vi "TestValid.vi"() -> ()   [LabVIEW 2023, in "HAF.lvlib"]
uses:
  HAF.lvlib
  DriverSetting/DriverSetting.lvclass
panel:
  out "error out":errorcluster
  out "Valid":bool
  out "DriverSetting Out":refnum<class "DriverSetting.lvclass">
  in  "error in (no error) 2":errorcluster
  in  "Type":string
  in  "DriverSetting In":refnum<class "DriverSetting.lvclass">
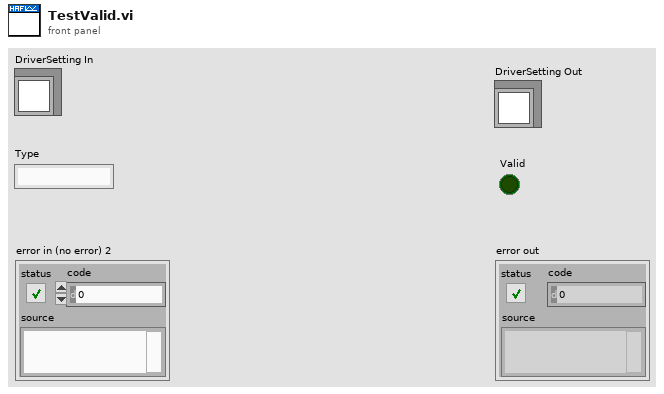
[diagram p1: front panel]
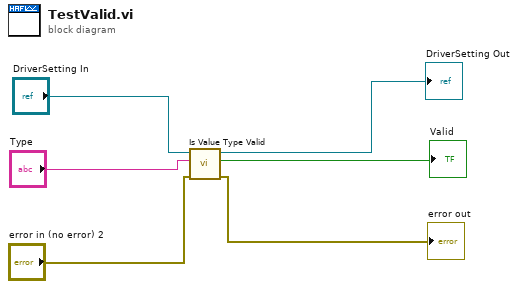
[diagram p0: block diagram]
diagram:
  n1 = call-dynamic "Is Value Type Valid.vi"("error in (no error)"="error in (no error) 2", "Value Type to Check"="Type", "DriverSetting in"="DriverSetting In") -> ("error out"=→"error out":errorcluster, "Is Valid"=→"Valid":bool, "DriverSetting out"=→"DriverSetting Out":refnum<class "DriverSetting.lvclass">)  [unwired: 6 in]
